vi "POSITIVE AND NEGATIVE USING FOR LOOP AND ARRAYS.vi"() -> ()   [LabVIEW 2018]
panel:
  out "NEGATIVE":i32[](array[numeric])
  out "POSITIVE":i32[](array[numeric])
  in  "INPUT":i32[](array[numeric])
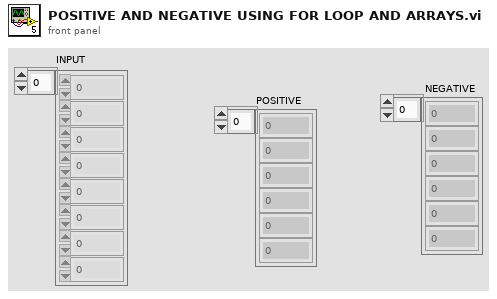
[diagram p1: front panel]
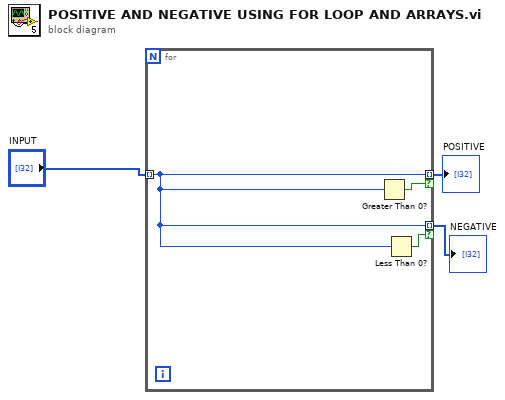
[diagram p0: block diagram]
diagram:
  n1 = for {
    tunnel: "INPUT" -> [w4] mode=indexing
    tunnel: [w4] -> w2 mode=indexing if=w6
    tunnel: [w4] -> w1 mode=indexing if=w5
    n2 = Greater Than 0?(x=w4) -> (x > 0?=w6:bool)
    n3 = Less Than 0?(x=w4) -> (x < 0?=w5:bool)
  }
  "POSITIVE" <- w2
  "NEGATIVE" <- w1
